vi "Unregister.vi"(8 "error in (no error)":errorcluster, 10 "Service":T1, 11 "MicronCLI in":refnum<class "MicronCLI.lvclass">) -> (0 "error out":errorcluster, 3 "MicronCLI out":refnum<class "MicronCLI.lvclass">)   [LabVIEW 2019, in "MicronCLI.lvclass"]
uses:
  MicronCLI.lvclass
  Typedefs/ServiceDetails.ctl
  MicronCLI.lvclass/MicronCLI.ctl
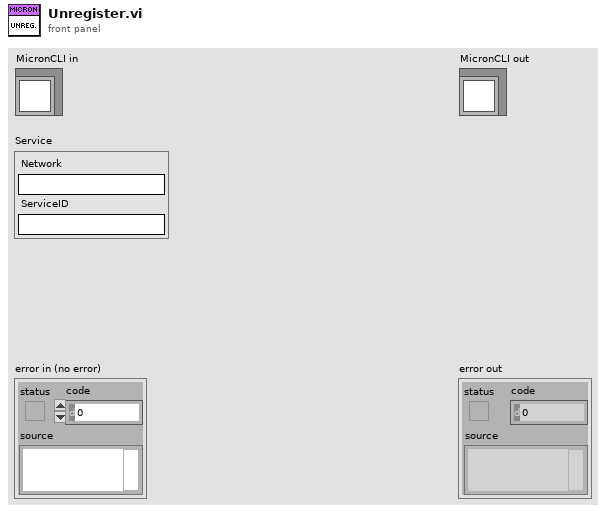
[diagram p1: front panel]
types:
  T1 = typedef "MicronCLI.lvclass/ServiceDetails.ctl" = cluster{"Network":string, "ServiceID":string}
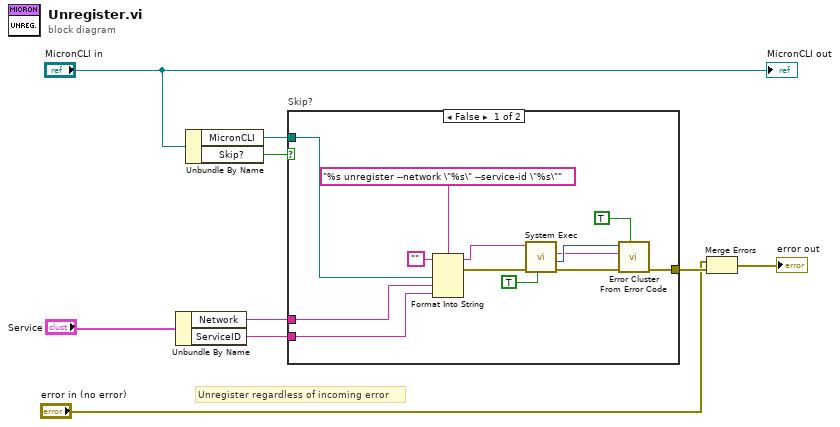
[diagram p0: block diagram]
diagram:
  # "Unregister regardless of incoming error"
  n1 = Unbundle By Name("Service") -> ("Network"=w4:string, "ServiceID"=w3:string)
  n2 = Unbundle By Name("MicronCLI in") -> ("MicronCLI"=w6:path, "Skip?"=w5:bool)
  n3 = case "Skip?" shown="False" w5 {
    tunnel: w6 -> [w19 _]
    tunnel: [w15 _] -> w9
    tunnel: w4 -> [w11 _]
    tunnel: w3 -> [w10 _]
    frame False {
      n4 = Format Into String(format string="%s unregister --network \"%s\" --service-id \"%s\"", initial string="", w19, w11, w10) -> (resulting string=w17:string, error out=w21:errorcluster)  [unwired: 1 in]
      n5 = call <vilib>:"System Exec.vi"("run minimized? (F)"=TRUE, "error in (no error)"=w21, "command line"=w17) -> ("error out"=w22:errorcluster, "return code"=w14:i32, "standard error"=w13:string)  [unwired: 5 in, 1 out]
      n6 = call <vilib>:"Error Cluster From Error Code.vi"("show call chain? (False)"=TRUE, "error in (no error)"=w22, "error message (\"\")"=w13, "error code (0)"=w14) -> ("error out"=w15:errorcluster)  [unwired: 5 in]
    }
    frame True {
    }
  }
  n7 = Merge Errors("error in (no error)", w9) -> (→"error out":errorcluster)
  "MicronCLI out" <- "MicronCLI in"
